vi "sub_vi_write_tsv_file.vi"(8 "error in (no error)":errorcluster, 10 "1D data":dbl[](array[numeric])) -> (0 "error out":errorcluster)   [LabVIEW 2019]
uses:
  <vilib>/Utility/file.llb/Write Delimited Spreadsheet (DBL).vi
panel:
  out "Path":string
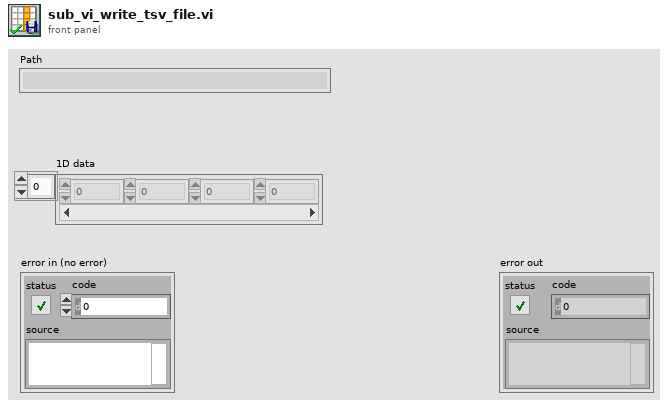
[diagram p1: front panel]
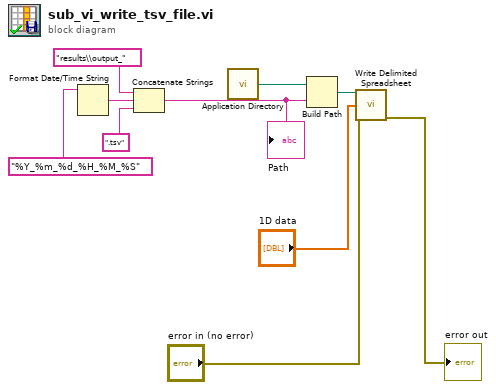
[diagram p0: block diagram]
diagram:
  n1 = Format Date/Time String(time format string (%c)="%Y_%m_%d_%H_%M_%S") -> (date/time string=w6:string)  [unwired: 2 in]
  n2 = Concatenate Strings("results\\output_" ("string"), w6, ".tsv" ("string")) -> (w8:string)
  "Path" <- w8
  n3 = call <vilib>:"Application Directory.vi"() -> ("Application Directory"=w9:path)
  n4 = Build Path(base path=w9, name or relative path=w8) -> (appended path=w10:path)
  n5 = call-poly <vilib>:"Write Delimited Spreadsheet.vi"("file path (dialog if empty)"=w10, "1D data"="1D data", "error in (no error)"="error in (no error)") -> ("error out"=→"error out":errorcluster)  [unwired: 11 in, 1 out]
